vi "Set Sciscan Scope Image Refresh.vi"(8 "error in":errorcluster, 10 "display every n-th frame":i8=10, 11 "GFG Refnum":refnum<vi>) -> (0 "error out":errorcluster, 3 "GFG Refnum Out":refnum<vi>)   [LabVIEW 2012, in "Sciscan Scope Daemon.lvlib"]
uses:
  Sciscan Scope Daemon.lvlib
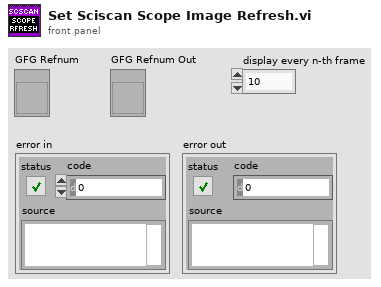
[diagram p1: front panel]
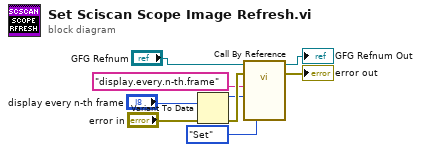
[diagram p0: block diagram]
diagram:
  n1 = Variant To Data(error in="error in", type="display every n-th frame", Variant="display every n-th frame") -> (data=w8:i8, error out=w9:errorcluster)
  n2 = call-by-ref "?"(reference="GFG Refnum", error in=w9, "Variable Name in"="display.every.n-th.frame", "Variant in"=w8, "Action"=enum16{"Init", "Set", "Get"}."Set") -> (reference out=→"GFG Refnum Out":refnum<vi>, error out=→"error out":errorcluster)  [unwired: 10 in, 7 out]
